vi "ToolBarButtonDraw_Escape.vi"(6 "Color":u32(colorbox), 8 "error in":errorcluster, 9 "rect":T1, 10 "Pict IN":picture, 11 "Gviewer in":refnum<class "Gviewer.lvclass">) -> (0 "error out":errorcluster, 2 "Pict OUT":picture, 3 "Gviewer out":refnum<class "Gviewer.lvclass">)   [LabVIEW 2020, in "Gviewer.lvclass"]
doc: "Press Escape button in toolbar"
uses:
  Gviewer.lvclass
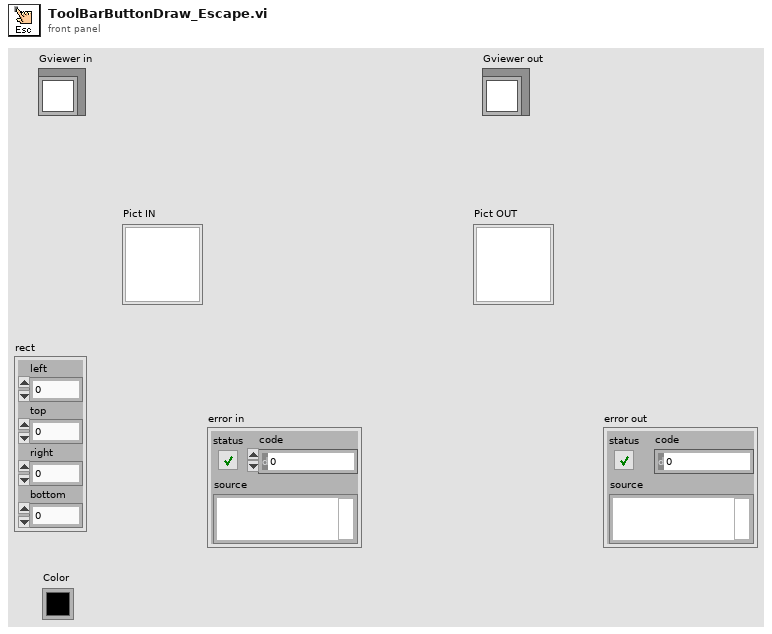
[diagram p1: front panel]
types:
  T1 = cluster{"left":i16, "top":i16, "right":i16, "bottom":i16}
  T2 = cluster{"horizontal":enum16{"left", "center", "right"}, "vertical":enum16{"top", "center", "bottom"}}
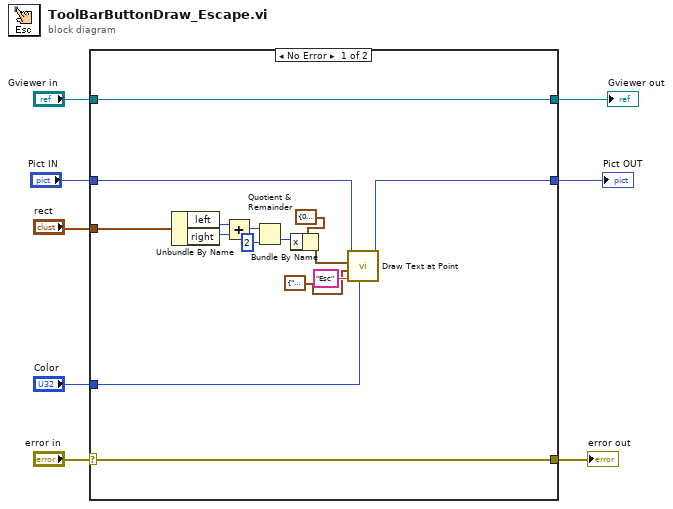
[diagram p0: block diagram]
diagram:
  n1 = case shown="No Error" "error in" {
    selector: "error in" -> [w10 w26]
    tunnel: "rect" -> [w14 _]
    tunnel: "Pict IN" -> [w13 w24]
    tunnel: [w12 w24] -> w6
    tunnel: "Color" -> [w11 _]
    tunnel: [w10 w26] -> w3
    tunnel: "Gviewer in" -> [w9 w25]
    tunnel: [w9 w25] -> w1
    frame No Error {
      n2 = Unbundle By Name(w14) -> ("left"=w20:i16, "right"=w21:i16)
      n3 = Add(x=w20, y=w21) -> (x+y=w22:i16)
      n4 = Quotient & Remainder(x=w22, y=i16 2) -> (floor(x/y)=w23:i16)  [unwired: 1 out]
      n5 = Bundle By Name(cluster=cluster{"x":i16, "y":i16} {"x"=0, "y"=13} ("origin"), "x"=w23) -> (w19:cluster{"x":i16, "y":i16})
      n6 = call <vilib>:"Draw Text at Point.vi"("text color(black)"=w11, "text"="Esc", "alignment(left, top)"=T2 {"horizontal"=enum."center", "vertical"=enum."center"}, "origin"=w19, "picture"=w13) -> ("new picture"=w12:picture)  [unwired: 5 in, 1 out]
    }
    frame Error {
    }
  }
  "Pict OUT" <- w6
  "Gviewer out" <- w1
  "error out" <- w3
